vi "Connect Meas Plugin APIs - Multiple Converter.vi"(0 "logic vi ref":refnum<vi>, 5 "sub vis":refnum<vi>[](array[refnum]), 11 "error in":errorcluster) -> (15 "error out":errorcluster)   [LabVIEW 2021, in "Converter.lvlib"]
uses:
  Converter.lvlib
  Converter Reusables/Converter Reusables.lvlib
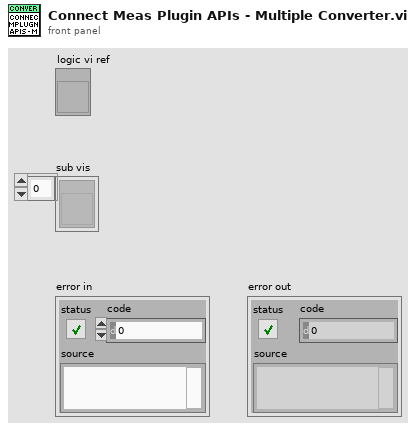
[diagram p1: front panel]
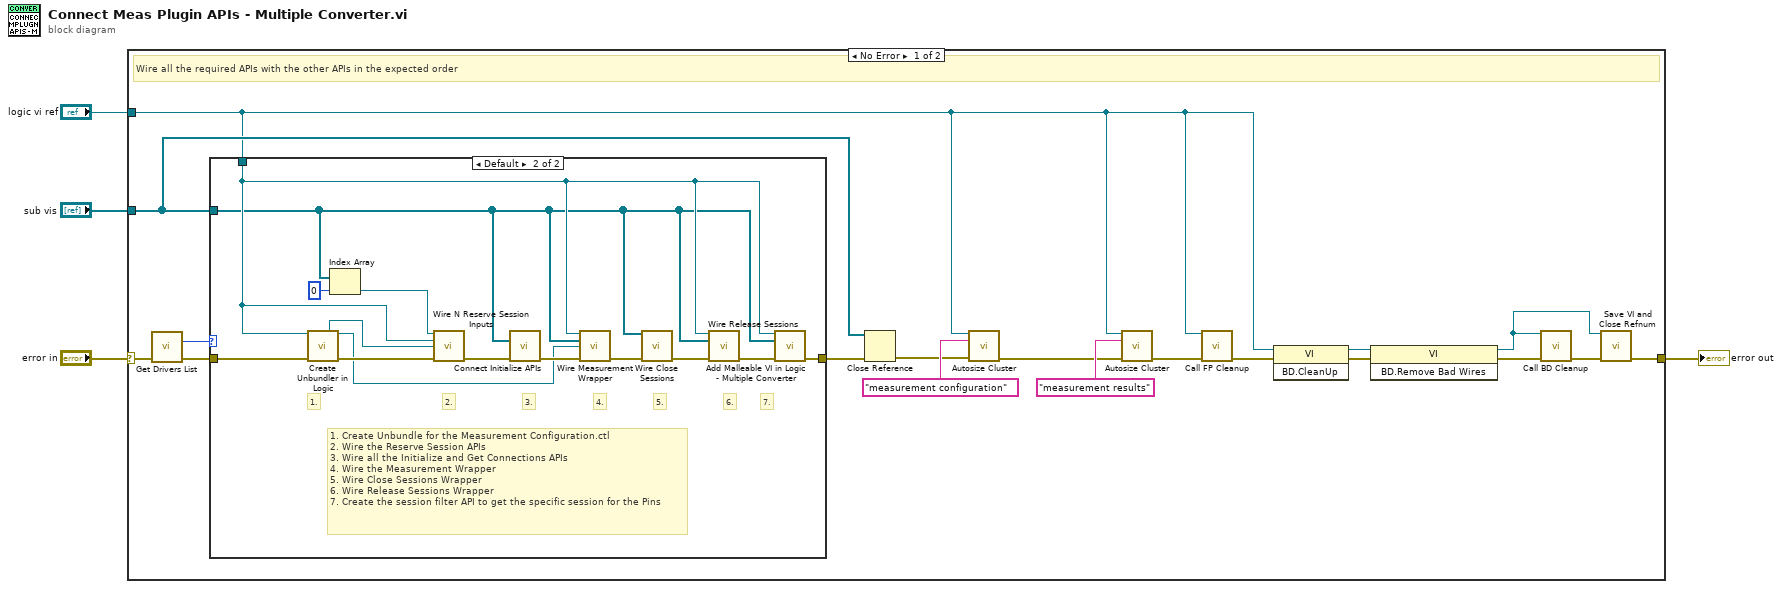
[diagram p0: block diagram]
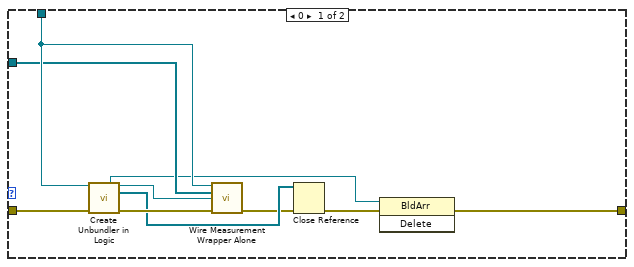
[diagram p2: hidden frame]
diagram:
  n1 = case shown="No Error" "error in" {
    selector: "error in" -> [w21 w46]
    tunnel: "logic vi ref" -> [w6 _]
    tunnel: "sub vis" -> [w17 _]
    tunnel: [w20 w46] -> w1
    frame No Error {
      # "Wire all the required APIs with the other APIs in the expected order"
      n2 = call "Get Drivers List.vi"() -> ("total driver list"=w15:i32)  [unwired: 10 in, 5 out]
      n3 = case shown="Default" w15 {
        tunnel: w21 -> [w30 w45]
        tunnel: w6 -> [w28 w33]
        tunnel: [w25 w34] -> w18
        tunnel: w17 -> [w27 w32]
        frame 0 {
          n4 = call "Create Unbundler in Logic.vi"("vi in"=w28, "error in"=w30) -> ("build array ref"=w26:refnum<vi>, "configration terminal"=w31:refnum<vi>, "unbundle output terms[]"=w24:refnum<vi>[], "error out"=w29:errorcluster)  [unwired: 10 in]
          n5 = call "Wire Measurement Wrapper Alone.vi"("vi reference"=w28, "sub vi in"=w27, "terminal"=w31, "error in"=w29) -> ("error out"=w22:errorcluster)  [unwired: 11 in]
          n6 = Close Reference(reference=w24, error in (no error)=w22) -> (error out=w23:errorcluster)
          n7 = invoke class="BldArr" method="Delete"(reference=w26, error in=w23) -> (error out=w25:errorcluster)  [unwired: 1 in, 2 out]
        }
        frame Default {
          # "1. Create Unbundle for the Measurement Configuration.ctl\n2. Wire the Reserve Session APIs\n3. Wire all the Initialize and Get Connections APIs\n4. Wire the Measurement Wrapper\n5. Wire Close Sessions Wrapper\n6. Wire Release Sessions Wrapper\n7. Create the session filter API to get the specific session for the Pins"
          # "7."
          # "6."
          # "5."
          # "4."
          # "3."
          # "2."
          # "1."
          n8 = call "Create Unbundler in Logic.vi"("vi in"=w33, "error in"=w45) -> ("build array ref"=w41:refnum<vi>, "configration terminal"=w37:refnum<vi>, "error out"=w42:errorcluster)  [unwired: 10 in, 1 out]
          n9 = Index Array(array=w32, index=0) -> (element=w43:refnum<vi>)
          n10 = call "Wire N Reserve Session Inputs.vi"("sub vi in"=w43, "vi reference"=w33, "build array"=w41, "error in"=w42) -> ("error out"=w36:errorcluster)  [unwired: 11 in]
          n11 = call "Connect Initialize APIs.vi"("sub vis"=w32, "error in"=w36) -> ("error out"=w40:errorcluster)  [unwired: 13 in]
          n12 = call "Wire Measurement Wrapper.vi"("vi reference"=w33, "sub vi in"=w32, "terminal"=w37, "error in"=w40) -> ("error out"=w39:errorcluster)  [unwired: 11 in]
          n13 = call "Wire Close Sessions.vi"("sub vis ref"=w32, "error in"=w39) -> ("error out"=w38:errorcluster)  [unwired: 13 in]
          n14 = call "Wire Release Sessions.vi"("logiv vi ref"=w33, "sub vis ref"=w32, "error in"=w38) -> ("error out"=w35:errorcluster)  [unwired: 12 in]
          n15 = call "Add Malleable VI in Logic - Multiple Converter.vi"("logic vi"=w33, "sub vis ref"=w32, "error in"=w35) -> ("error out"=w34:errorcluster)  [unwired: 12 in]
        }
      }
      n16 = Close Reference(reference=w17, error in (no error)=w18) -> (error out=w10:errorcluster)
      n17 = call "Autosize Cluster.vi"("vi refnum"=w6, "name"="measurement configuration" ("name/order"), "error in"=w10) -> ("error out"=w8:errorcluster)  [unwired: 12 in]
      n18 = call "Autosize Cluster.vi"("vi refnum"=w6, "name"="measurement results" ("name/order"), "error in"=w8) -> ("error out"=w7:errorcluster)  [unwired: 12 in]
      n19 = call "Call FP Cleanup.vi"("vi"=w6, "error in"=w7) -> ("error out"=w19:errorcluster)  [unwired: 13 in]
      n20 = invoke class="VI" method="BD.CleanUp"(reference=w6, error in=w19) -> (reference out=w14:refnum<vi>, error out=w12:errorcluster)  [unwired: 1 in, 1 out]
      n21 = invoke class="VI" method="BD.Remove Bad Wires"(reference=w14, error in=w12) -> (reference out=w5:refnum<vi>, error out=w13:errorcluster)  [unwired: 1 in, 1 out]
      n22 = call "Call BD Cleanup.vi"("vi"=w5, "error in"=w13) -> ("error out"=w16:errorcluster)  [unwired: 13 in]
      n23 = call "Save VI and Close Refnum.vi"("vi refnum"=w5, "error in"=w16) -> ("error out"=w20:errorcluster)  [unwired: 13 in]
    }
    frame Error {
    }
  }
  "error out" <- w1
